vi "SA_GET_MARKER.vi"(4 "Units":i64(ring) items=["Hz"=1, "KHz"=1000, "MHz"=1000000, "GHz"=1000000000], 5 "offset":dbl, 6 "Set MKR Freq ()":dbl=2000000.0 format="%#_13g", 7 "Use PK Search (T)":bool=TRUE, 8 "error in":errorcluster {"code" format="%.0x"}, 10 "IsPSA?(t)":bool, 11 "Session In":refnum<visa-resource-name>="TCPIP0::169.254.70.120::inst0::INSTR") -> (0 "error out":errorcluster {"code" format="%.0x"}, 1 "Ampl_corr":dbl=-76.918, 2 "Mark Values":dbl[](array[numeric])=[40000.0232, -76.918], 3 "Session Out":refnum<visa-resource-name>="TCPIP0::169.254.70.120::inst0::INSTR")   [LabVIEW 2018]
doc: "Launches the Instrument I/O Assistant, which you can use to communicate with message-based instruments and graphically parse the response. For example you can communicate with an instrument that uses a serial, Ethernet, or GPIB interface."
uses:
  Initialize References/Station References Global.vi
panel:
  out "Numeric":i32
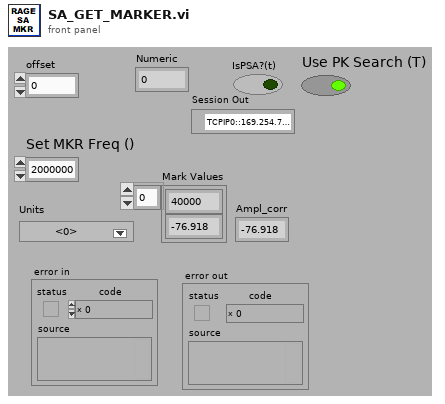
[diagram p1: front panel]
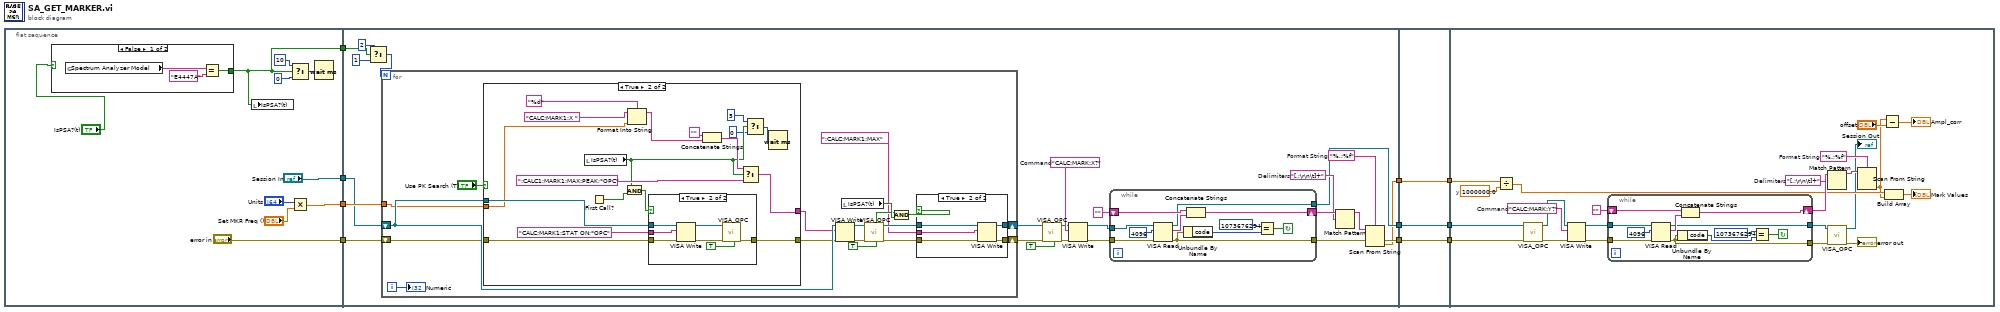
[diagram p0: block diagram]
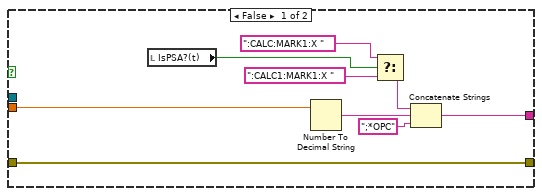
[diagram p4: hidden frame]
diagram:
  n1 = flat-sequence {
    tunnel: ["error in"] -> w4
    tunnel: ["Session In"] -> w3
    tunnel: [w17] -> w2
    tunnel: [w12] -> w1
    tunnel: [w41] -> w10
    tunnel: [w40] -> w8
    tunnel: [w39] -> w6
    tunnel: w4 -> [w31]
    tunnel: w3 -> [w35]
    tunnel: w2 -> [w38]
    tunnel: w1 -> [w27]
    tunnel: w10 -> [w122]
    tunnel: [w122] -> w9
    tunnel: w8 -> [w121]
    tunnel: [w121] -> w7
    tunnel: w6 -> [w120]
    tunnel: [w120] -> w5
    tunnel: w9 -> [w130]
    tunnel: w7 -> [w128]
    tunnel: w5 -> [w136]
    frame #0 {
      n2 = case shown="False" "IsPSA?(t)" {
        selector: "IsPSA?(t)" -> [_ w24]
        tunnel: [w21 w24] -> w12
        frame False {
          n3 = global read "Station References Global.vi" "Spectrum Analyzer Model"() -> (w23:string)
          n4 = Equal?(x=w23, y="E4447A") -> (x = y?=w21:bool)
        }
        frame True {
        }
      }
      n5 = local write "IsPSA?(t)"(w12) -> ()
      n6 = Select(t=u32 10 ("milliseconds to wait"), s=w12, f=u32 0) -> (s? t:f=w15:u32)
      n7 = Multiply(x="Units", y="Set MKR Freq ()") -> (x*y=w17:dbl)
      n8 = Wait (ms)(milliseconds to wait=w15) -> ()  [unwired: 1 out]
    }
    frame #1 {
      w42 = "[,;\r\n\t]+"  # Delimiters
      w43 = "%.;%f"  # Format String
      w46 = "CALC:MARK:X?"  # Command
      n9 = Select(t=2, s=w27, f=1) -> (s? t:f=w28:i32)
      n10 = for {
        N: w28 -> [_]
        tunnel: w38 -> [w49]
        shift-right: [w61] -> w30
        shift-left: w35 -> [w65]
        shift-right: [w60] -> w29
        shift-left: w31 -> [w63]
        i -> [w52]
        n11 = case shown="True" "Use PK Search (T)" {
          tunnel: [w80 w100] -> w62
          tunnel: w65 -> [_ w97]
          tunnel: [w79 w95] -> w64
          tunnel: w63 -> [w79 w94]
          tunnel: w49 -> [w74 w90]
          frame False {
            n12 = local read "IsPSA?(t)"() -> (w76:bool)
            n13 = Number To Decimal String(number=w74) -> (decimal integer string=w82:string)  [unwired: 1 in]
            n14 = Select(t=":CALC:MARK1:X " ("StaticText"), s=w76, f=":CALC1:MARK1:X " ("StaticText")) -> (s? t:f=w75:string)
            n15 = Concatenate Strings(w75, w82, ";*OPC" ("string")) -> (w80:string)
          }
          frame True {
            n16 = local read "IsPSA?(t)"() -> (w88:bool)
            n17 = First Call?() -> (First Call?: T/F=w93:bool)
            n18 = And(x=w88, y=w93) -> (x .and. y?=w92:bool)
            n19 = Format Into String(format string="%d", initial string="CALC:MARK1:X " ("StaticText"), w90) -> (resulting string=w83:string)  [unwired: 1 in, 1 out]
            n20 = case shown="True" w92 {
              tunnel: "CALC:MARK1:STAT ON;*OPC" ("StaticText") -> [_ w108]
              tunnel: w97 -> [_ w107]
              tunnel: [w101 w103] -> w95
              tunnel: w94 -> [w101 w102]
              frame False {
              }
              frame True {
                n21 = VISA Write(VISA resource name=w107, write buffer=w108, error in (no error)=w102) -> (VISA resource name out=w106:refnum<visa-resource-name>, error out=w105:errorcluster)  [unwired: 1 out]
                n22 = call "VISA_OPC.vi"("OPC(T)"=TRUE, "error in"=w105, "Session In"=w106) -> ("error out"=w103:errorcluster)  [unwired: 6 in, 2 out]
              }
            }
            n23 = Concatenate Strings("", w83) -> (w96:string)
            n24 = Select(t=w96, s=w88, f=":CALC1:MARK1:MAX:PEAK;*OPC" ("StaticText")) -> (s? t:f=w100:string)
            n25 = Select(t=u32 5 ("milliseconds to wait"), s=w88, f=u32 0) -> (s? t:f=w86:u32)
            n26 = Wait (ms)(milliseconds to wait=w86) -> ()  [unwired: 1 out]
          }
        }
        n27 = VISA Write(VISA resource name=w65, write buffer=w62, error in (no error)=w64) -> (VISA resource name out=w58:refnum<visa-resource-name>, error out=w57:errorcluster)  [unwired: 1 out]
        n28 = local read "IsPSA?(t)"() -> (w59:bool)
        n29 = call "VISA_OPC.vi"("OPC(T)"=TRUE, "error in"=w57, "Session In"=w58) -> ("error out"=w56:errorcluster, "Session Out"=w55:refnum<visa-resource-name>, "OPC?(T)"=w54:bool)  [unwired: 6 in]
        n30 = And(x=w54, y=w59) -> (x .and. y?=w50:bool)
        n31 = case shown="True" w50 {
          tunnel: w55 -> [w68 w73]
          tunnel: ":CALC:MARK1:MAX" ("StaticText") -> [_ w72]
          tunnel: [w68 w71] -> w61
          tunnel: [w67 w70] -> w60
          tunnel: w56 -> [w67 w69]
          frame False {
          }
          frame True {
            n32 = VISA Write(VISA resource name=w73, write buffer=w72, error in (no error)=w69) -> (VISA resource name out=w71:refnum<visa-resource-name>, error out=w70:errorcluster)  [unwired: 1 out]
          }
        }
        "Numeric" <- w52
      }
      n33 = call "VISA_OPC.vi"("OPC(T)"=TRUE, "error in"=w29, "Session In"=w30) -> ("error out"=w33:errorcluster, "Session Out"=w34:refnum<visa-resource-name>)  [unwired: 6 in, 1 out]
      n34 = VISA Write(VISA resource name=w34, write buffer=w46, error in (no error)=w33) -> (VISA resource name out=w37:refnum<visa-resource-name>, error out=w36:errorcluster)  [unwired: 1 out]
      n35 = while {
        tunnel: w37 -> [w116]
        shift-right: [w110] -> w45
        shift-left: "" -> [w115]
        tunnel: w36 -> [w113]
        tunnel: [w112] -> w48
        tunnel: [w109] -> w40
        stop <- w111 continue-if-true
        n36 = VISA Read(VISA resource name=w116, byte count=u32 4096 ("byte count (0)"), error in (no error)=w113) -> (VISA resource name out=w109:refnum<visa-resource-name>, read buffer=w114:string, error out=w112:errorcluster)  [unwired: 1 out]
        n37 = Unbundle By Name(w112) -> ("code"=w118:i32)
        n38 = Concatenate Strings(w115, w114) -> (w110:string)
        n39 = Equal?(x=1073676294, y=w118) -> (x = y?=w111:bool)
      }
      n40 = Match Pattern(string=w45, regular expression=w42) -> (before substring=w44:string)  [unwired: 1 in, 3 out]
      n41 = Scan From String(format string=w43, input string=w44, error in=w48) -> (error out=w41:errorcluster, output 1=w39:dbl)  [unwired: 2 in, 2 out]
    }
    frame #2 {
    }
    frame #3 {
      w134 = 1000000.0  # y
      w140 = "[,;\r\n\t]+"  # Delimiters
      w139 = "%.;%f"  # Format String
      w137 = "CALC:MARK:Y?"  # Command
      n42 = Divide(x=w136, y=w134) -> (x/y=w135:dbl)
      n43 = call "VISA_OPC.vi"("error in"=w130, "Session In"=w128) -> ("error out"=w129:errorcluster, "Session Out"=w127:refnum<visa-resource-name>)  [unwired: 7 in, 1 out]
      n44 = VISA Write(VISA resource name=w127, write buffer=w137, error in (no error)=w129) -> (VISA resource name out=w141:refnum<visa-resource-name>, error out=w142:errorcluster)  [unwired: 1 out]
      n45 = while {
        tunnel: w141 -> [w153]
        shift-right: [w147] -> w143
        shift-left: "" -> [w152]
        tunnel: w142 -> [w150]
        tunnel: [w149] -> w126
        tunnel: [w146] -> w124
        stop <- w148 continue-if-true
        n46 = VISA Read(VISA resource name=w153, byte count=u32 4096 ("byte count (0)"), error in (no error)=w150) -> (VISA resource name out=w146:refnum<visa-resource-name>, read buffer=w151:string, error out=w149:errorcluster)  [unwired: 1 out]
        n47 = Unbundle By Name(w149) -> ("code"=w155:i32)
        n48 = Concatenate Strings(w152, w151) -> (w147:string)
        n49 = Equal?(x=1073676294, y=w155) -> (x = y?=w148:bool)
      }
      n50 = Match Pattern(string=w143, regular expression=w140) -> (before substring=w144:string)  [unwired: 1 in, 3 out]
      n51 = call "VISA_OPC.vi"("error in"=w126, "Session In"=w124) -> ("error out"=→"error out":errorcluster, "Session Out"=→"Session Out":refnum<visa-resource-name>)  [unwired: 7 in, 1 out]
      n52 = Scan From String(format string=w139, input string=w144) -> (output 1=w132:dbl)  [unwired: 3 in, 3 out]
      n53 = Subtract(x=w132, y="offset") -> (x-y=→"Ampl_corr":dbl)
      n54 = Build Array(w135, w132) -> (→"Mark Values":dbl[])
    }
  }
